vi "Call_Pre_Analysis_An_Plugin.vi"(2 "Analogue In":dbl[][](array[numeric]), 3 "Plugin Name":string) -> (0 "Analogue Out":dbl[][](array[numeric]))   [LabVIEW 2010]
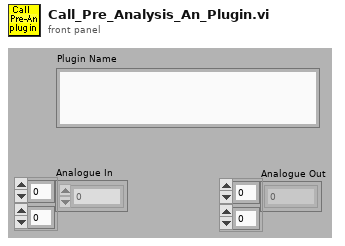
[diagram p1: front panel]
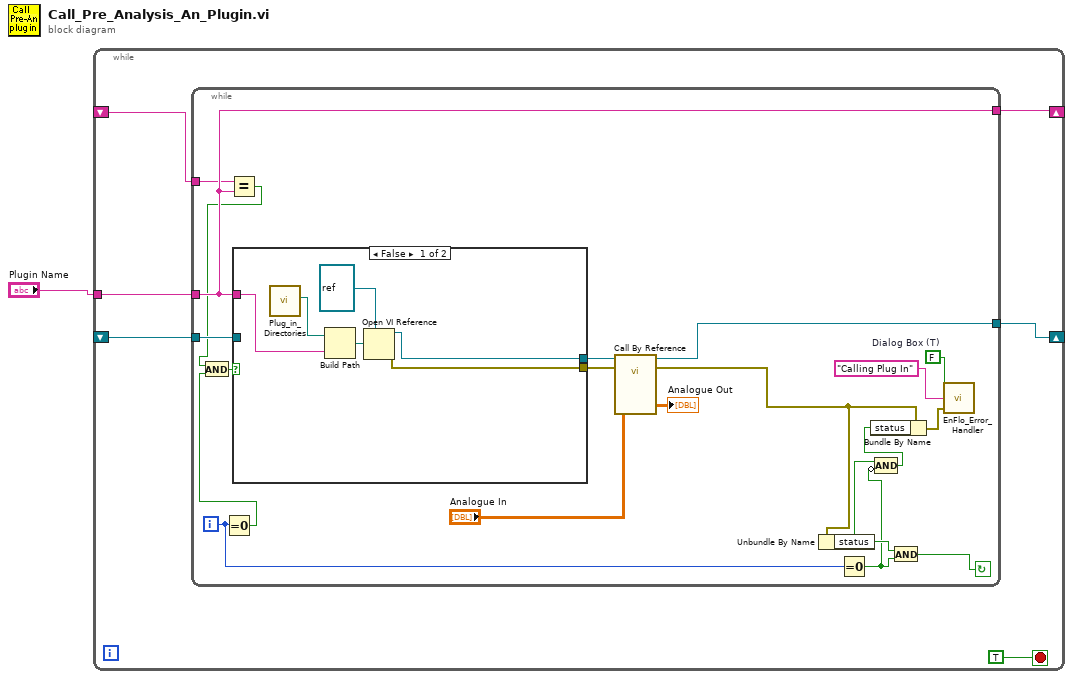
[diagram p0: block diagram]
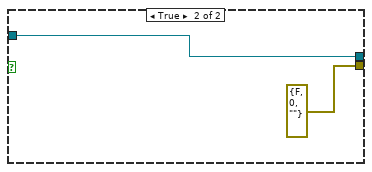
[diagram p2: hidden frame]
diagram:
  n1 = while {
    tunnel: "Plugin Name" -> [w7]
    shift-right: [w6] -> _
    shift-left: _ -> [w5]
    shift-right: [w3] -> _
    shift-left: _ -> [w2]
    stop <- TRUE stop-if-true
    n2 = while {
      tunnel: w7 -> [w14]
      tunnel: [w25] -> w6
      tunnel: w5 -> [w24]
      tunnel: [w14] -> w3
      tunnel: w2 -> [w13]
      i -> [w15]
      stop <- w21 continue-if-true
      w23 = FALSE  # Dialog Box (T)
      n3 = Equal To 0?(x=w15) -> (x = 0?=w11:bool)
      n4 = Equal?(x=w13, y=w14) -> (x = y?=w10:bool)
      n5 = And(x=w10, y=w11) -> (x .and. y?=w12:bool)
      n6 = case shown="False" w12 {
        tunnel: [w28 errorcluster {"status"=FALSE, "code"=0, "source"=""} ("error out")] -> w27
        tunnel: [w29 w34] -> w26
        tunnel: w14 -> [w32 _]
        tunnel: w24 -> [_ w34]
        frame False {
          n7 = call "Plug_in_Directories.vi"() -> ("Pre_Analysis_Analogue_Plugins"=w31:path)  [unwired: 3 out]
          n8 = Build Path(base path=w31, name or relative path=w32) -> (appended path=w33:path)
          n9 = Open VI Reference(type specifier VI Refnum (for type only)=refnum<vi> refnum, vi path=w33) -> (vi reference=w29:refnum<vi>, error out=w28:errorcluster)  [unwired: 2 in, 2 out]
        }
        frame True {
        }
      }
      n10 = call-by-ref "?"(reference=w26, error in=w27, "Analogue In"="Analogue In") -> (reference out=w25:refnum<vi>, error out=w20:errorcluster, "Analogue Out"=→"Analogue Out":dbl[][])  [unwired: 10 in]
      n11 = Unbundle By Name(w20) -> ("status"=w18:bool)
      n12 = Equal To 0?(x=w15) -> (x = 0?=w17:bool)
      n13 = Compound Arithmetic op=AND(w18, invert w17) -> (w16:bool)
      n14 = Bundle By Name(cluster=w20, "status"=w16) -> (w19:errorcluster)
      n15 = And(x=w18, y=w17) -> (x .and. y?=w21:bool)
      n16 = call "EnFlo_Error_Handler.vi"("error in (no error)"=w19, "Error Type"="Calling Plug In", "Dialog Box (T)"=w23) -> ()  [unwired: 3 out]
    }
  }
